vi "Create Text Object.vi"(8 "error in (no error)":errorcluster, 9 "Alpha":sgl=1.0, 10 "Color Box":u32(colorbox), 11 "Value String":string) -> (0 "error out":errorcluster, 1 "Numeric":sgl, 3 "Scene:New Object":refnum<vi>)   [LabVIEW 2020, in "3D Plot.lvclass"]
uses:
  <vilib>/Math Plots/3D Math Plots/3D Plot/3D Plot/3D Plot.lvclass
  <vilib>/picture/3D Picture Control/Object/Create Object (name).vi
  <vilib>/picture/3D Picture Control/NI_3D Picture Control.lvlib
  <vilib>/Math Plots/Plot Private Lib/NI_Math Plot Private Lib.lvlib
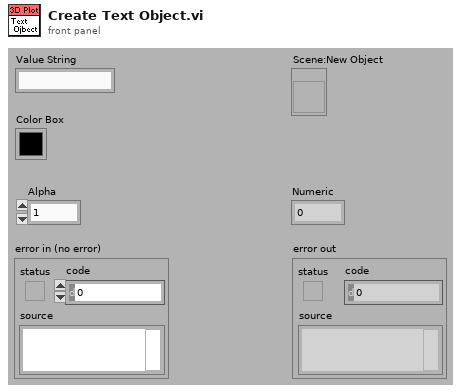
[diagram p1: front panel]
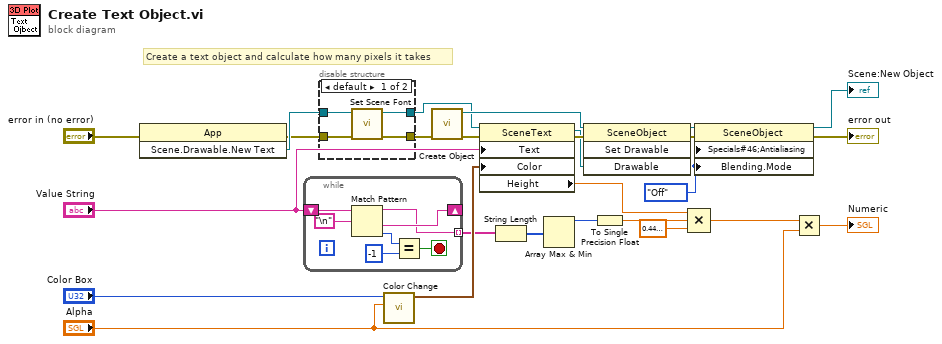
[diagram p0: block diagram]
diagram:
  w17 = enum16{"Inherit Value", "Off", "On"}."Off" ("Specials:Anti-aliasing")
  # "Create a text object and calculate how many pixels it takes"
  n1 = invoke class="App" method="Scene.Drawable.New Text"(error in="error in (no error)") -> (error out=w9:errorcluster, "Scene.Drawable.New Text"=w11:refnum<vi>)  [unwired: 2 in, 1 out]
  n2 = while {
    shift-right: [w32] -> _
    shift-left: "Value String" -> [w33]
    tunnel: [w31] -> w7 mode=indexing
    stop <- w29 stop-if-true
    n3 = Match Pattern(string=w33, regular expression="\n") -> (before substring=w31:string, after substring=w32:string, offset past match=w28:i32)  [unwired: 2 out]
    n4 = Equal?(x=w28, y=-1) -> (x = y?=w29:bool)
  }
  n5 = disable-structure shown="default" {
    disable-tunnel: [w37 w39] -> w12
    disable-tunnel: w11 -> [w36 w39]
    disable-tunnel: w9 -> [w35 w38]
    disable-tunnel: [w34 w38] -> w8
    frame condition #0 (active) {
      n6 = call <vilib>:"Set Scene Font.vi"("error in (no error)"=w35, "Scene Text Refnum"=w36) -> ("error out"=w34:errorcluster, "Dup Scene Text Refnum"=w37:refnum<vi>)  [unwired: 8 out]
    }
    frame condition #1 {
    }
  }
  n7 = call <vilib>:"Color Change.vi"("Alpha"="Alpha", "Color"="Color Box") -> ("RGBA"=w10:cluster{"R":sgl, "G":sgl, "B":sgl, "A":sgl})  [unwired: 9 out]
  n8 = call-poly <vilib>:"Create Object.vi"("error in (no error)"=w8) -> ("error out"=w16:errorcluster, "Scene:New Object"=w20:refnum<vi>)  [unwired: 9 in]
  n9 = property class="SceneText"(reference=w12, error in=w16, "Text"="Value String", "Color"=w10) -> (reference out=w13:refnum<vi>, error out=w15:errorcluster, "Height"=w4:sgl)
  n10 = String Length(string=w7) -> (length=w6:i32[])
  n11 = Array Max & Min(array=w6) -> (max value=w5:i32)  [unwired: 3 out]
  n12 = invoke class="SceneObject" method="Set Drawable"(reference=w20, error in=w15, "Drawable"=w13) -> (reference out=w19:refnum<vi>, error out=w18:errorcluster)  [unwired: 1 in, 2 out]
  n13 = To Single Precision Float(number=w5) -> (single precision float=w14:sgl)
  n14 = Compound Arithmetic op=MULTIPLY(w4, w14, sgl 0.45 ("y")) -> (w3:sgl)
  n15 = property class="SceneObject"(reference=w19, error in=w18, "Specials#46;Antialiasing"=w17, "Blending.Mode"=w17) -> (reference out=→"Scene:New Object":refnum<vi>, error out=→"error out":errorcluster)
  n16 = Multiply(x=w3, y="Alpha") -> (x*y=→"Numeric":sgl)
